vi "Create.vi"(8 "error in (no error)":errorcluster, 10 "Event Module Q":refnum<class "MessageQ.lvclass">, 11 "Core Module Q":refnum<class "MessageQ.lvclass">) -> (0 "error out":errorcluster, 3 "DebugHTTPController out":refnum<class "DebugHTTPController.lvclass">)   [LabVIEW 2020, in "Volatus.lvlib" / "DebugHTTPController.lvclass"]
uses:
  DebugHTTPController.lvclass
  MessageQ/MessageQ.lvclass
  DebugHTTPController.lvclass/DebugHTTPController.ctl
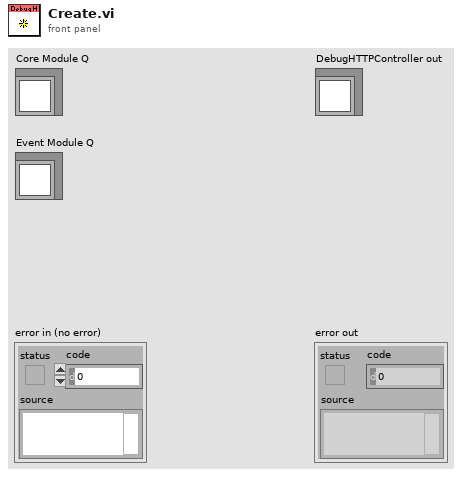
[diagram p1: front panel]
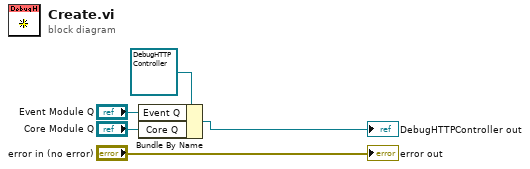
[diagram p0: block diagram]
diagram:
  n1 = Bundle By Name(cluster=refnum<class "DebugHTTPController.lvclass"> refnum ("DebugHTTPController in"), "Event Q"="Event Module Q", "Core Q"="Core Module Q") -> (→"DebugHTTPController out":refnum<class "DebugHTTPController.lvclass">)
  "error out" <- "error in (no error)"
